vi "Configure No-Operation-Pending Flag.vi"(8 "error in (no error)":errorcluster, 10 "No-operation-pending Flag (0: Include)":i32(ring) items=["Include", "Exclude"], 11 "VISA resource name":refnum<visa-resource-name>) -> (0 "error out":errorcluster, 3 "VISA resource name out":refnum<visa-resource-name>)   [LabVIEW 2019, in "Keithley 6517.lvlib"]
doc: "Controls the no-operation-pending flag in the internal process of determining whether all pending operations of an initiate command are completed.\n\n<B>Note:</B>\nThis VI is <B>NOT</B> compatible with model <B>6514</B>."
uses:
  Keithley 6517.lvlib
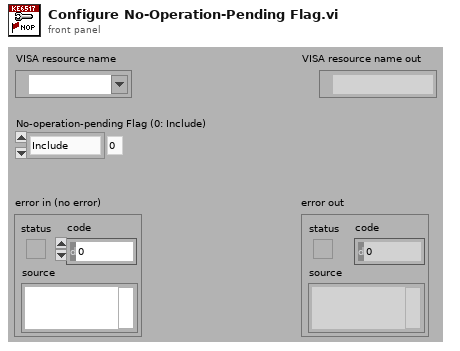
[diagram p1: front panel]
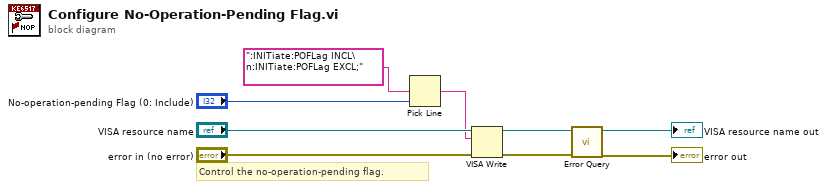
[diagram p0: block diagram]
diagram:
  # "Control the no-operation-pending flag."
  n1 = Pick Line(multi-line string=":INITiate:POFLag INCL\n:INITiate:POFLag EXCL;", line index="No-operation-pending Flag (0: Include)") -> (output string=w1:string)  [unwired: 1 in]
  n2 = VISA Write(VISA resource name="VISA resource name", write buffer=w1, error in (no error)="error in (no error)") -> (VISA resource name out=w7:refnum<visa-resource-name>, error out=w6:errorcluster)  [unwired: 1 out]
  n3 = call "Error Query.vi"("error in (no error)"=w6, "VISA resource name"=w7) -> ("error out"=→"error out":errorcluster, "VISA resource name out"=→"VISA resource name out":refnum<visa-resource-name>)  [unwired: 6 in, 2 out]
